vi "DEMO_07_OpenFuzhiMode.vi"() -> ()   [LabVIEW 2014]
uses:
  <vilib>/Instr/_visa.llb/VISA Configure Serial Port (Instr).vi
panel:
  in  "设置 3":bool
  in  "选择开关 3":u16(ring) items=["开始", "停止"]
  in  "选择开关 2":u16(ring) items=["开始", "停止"]
  in  "设置 2":bool
  in  "打开串口":bool
  in  "选择开关":u16(ring) items=["开始", "停止"]
  in  "上位机控制":bool
  in  "设置":bool
  in  "VISA资源名称":refnum<visa-resource-name>="COM1"
  in  "波特率":u32(ring)=9600 items=["75"=75, "110"=110, "134"=134, "150"=150, "300"=300, "600"=600, "1200"=1200, "1800"=1800, "2400"=2400, "4800"=4800, "7200"=7200, "9600"=9600, "14400"=14400, "19200"=19200, "28800"=28800, "38400"=38400, "56000"=56000, "57600"=57600, "115200"=115200, "128000"=128000, "230400"=230400]
  in  "奇偶":enum16{"None", "Odd", "Even", "Mark", "Space"}(ring) caption="校验"
  # "幅值校正控制开启"
  # "一路"
  # "二路"
  # "三路"
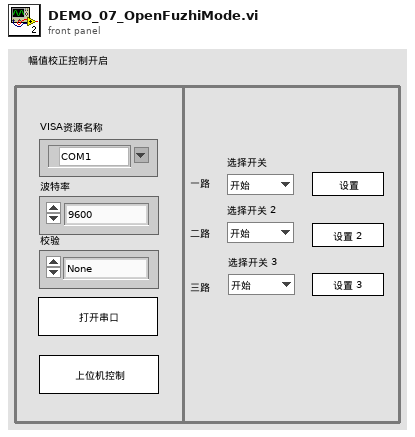
[diagram p1: front panel]
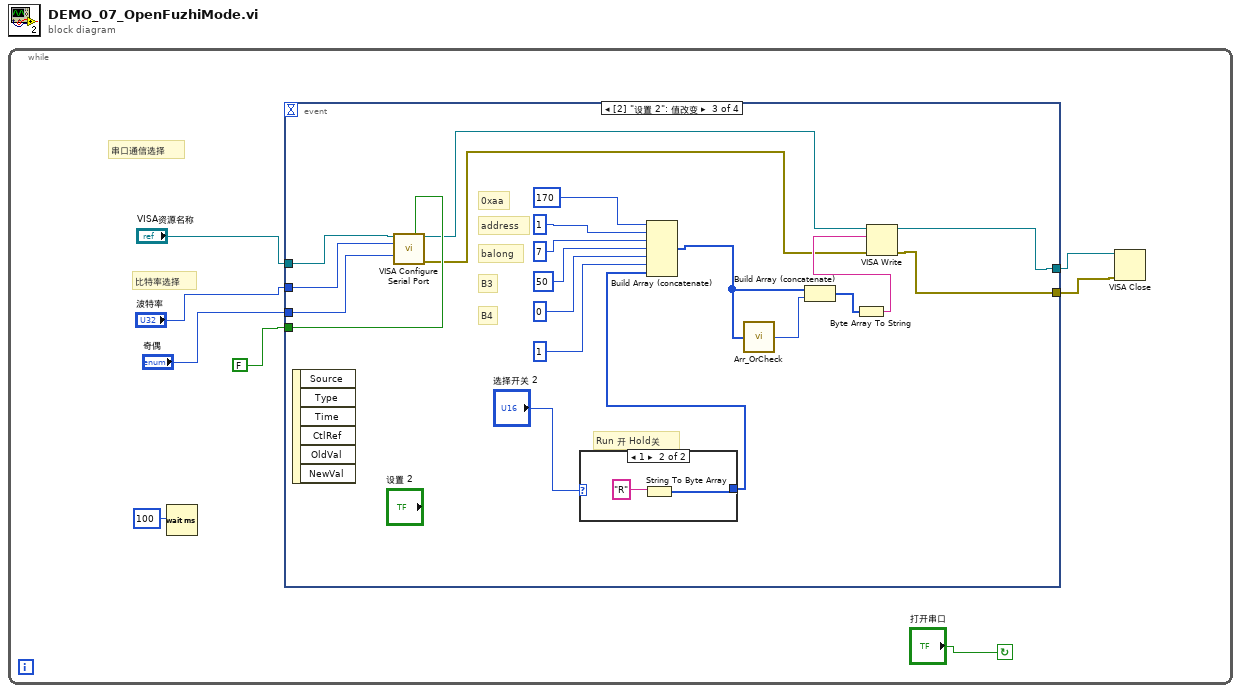
[diagram p0: block diagram]
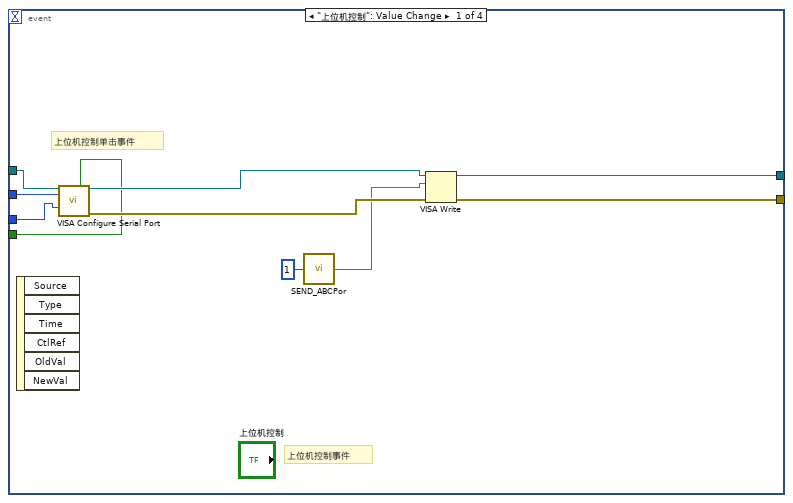
[diagram p2: hidden frame]
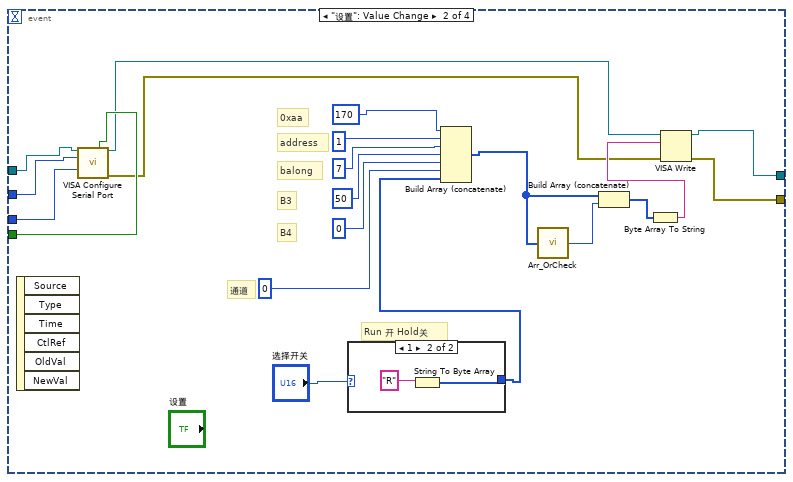
[diagram p3: hidden frame]
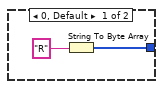
[diagram p4: hidden frame]
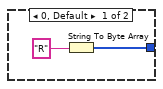
[diagram p5: hidden frame]
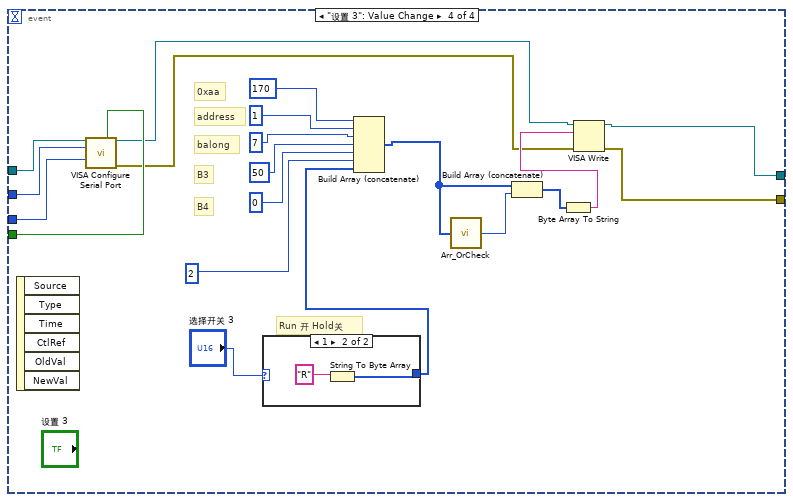
[diagram p6: hidden frame]
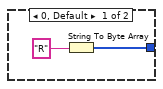
[diagram p7: hidden frame]
diagram:
  n1 = while {
    stop <- "打开串口" continue-if-true
    # "比特率选择"
    # "串口通信选择"
    n2 = Wait (ms)(milliseconds to wait=100) -> ()  [unwired: 1 out]
    n3 = event shown="[2] \"设置 2\": 值改变" {
      selector: _ -> [_ _ _ _]
      dyn-events: _ -> [_ _ _ _]
      timeout: _ -> [_ _ _ _]
      tunnel: "VISA资源名称" -> [w18 w38 w50 w76]
      tunnel: "波特率" -> [w17 w37 w49 w75]
      tunnel: "奇偶" -> [w16 w36 w48 w74]
      tunnel: [w13 w21 w44 w69] -> w1
      tunnel: [w12 w22 w43 w70] -> w6
      tunnel: FALSE -> [w11 w30 w47 w73]
      event "上位机控制": Value Change {
        # "上位机控制事件"
        # "上位机控制单击事件"
        n4 = event-data() -> ()  [unwired: 1 in, 6 out]
        n5 = call-poly "VISA Configure Serial Port"("VISA resource name"=w18, "Enable Termination\nChar (T)"=w11, "baud rate (9600)"=w17, "parity (0:none)"=w16) -> ("VISA resource name out"=w15:refnum<visa-resource-name>, "error out"=w14:errorcluster)  [unwired: 10 in]
        n6 = call "SEND_ABCPor.vi"("设备地址 1 开始"=1) -> ("输出字符串"=w9:string)
        n7 = VISA Write(VISA resource name=w15, write buffer=w9, error in (no error)=w14) -> (VISA resource name out=w13:refnum<visa-resource-name>, error out=w12:errorcluster)  [unwired: 1 out]
      }
      event "设置": Value Change {
        # "通道"
        # "B4"
        # "B3"
        # "Run 开 Hold关"
        # "balong"
        # "address"
        # "0xaa"
        n8 = event-data() -> ()  [unwired: 1 in, 6 out]
        n9 = call-poly "VISA Configure Serial Port"("VISA resource name"=w38, "Enable Termination\nChar (T)"=w30, "baud rate (9600)"=w37, "parity (0:none)"=w36) -> ("VISA resource name out"=w24:refnum<visa-resource-name>, "error out"=w23:errorcluster)  [unwired: 10 in]
        n10 = case shown="1" "选择开关" {
          tunnel: [w39 w41] -> w27
          frame 0, Default {
            n11 = String To Byte Array(string="R") -> (unsigned byte array=w39:u8[])
          }
          frame 1 {
            n12 = String To Byte Array(string="R") -> (unsigned byte array=w41:u8[])
          }
        }
        n13 = Build Array (concatenate)(170, 1, 7, 50, 0, 0 ("元素"), w27) -> (w26:i32[])
        n14 = call "Arr_OrCheck.vi"("数组"=w26) -> ("抑或的数据值"=w32:u8)
        n15 = Build Array (concatenate)(w26, w32) -> (w31:i32[])
        n16 = Byte Array To String(unsigned byte array=w31) -> (string=w25:string)
        n17 = VISA Write(VISA resource name=w24, write buffer=w25, error in (no error)=w23) -> (VISA resource name out=w21:refnum<visa-resource-name>, error out=w22:errorcluster)  [unwired: 1 out]
      }
      event "设置 2": Value Change {
        # "Run 开 Hold关"
        # "B4"
        # "B3"
        # "balong"
        # "address"
        # "0xaa"
        n18 = event-data() -> ()  [unwired: 1 in, 6 out]
        n19 = call-poly "VISA Configure Serial Port"("VISA resource name"=w50, "Enable Termination\nChar (T)"=w47, "baud rate (9600)"=w49, "parity (0:none)"=w48) -> ("VISA resource name out"=w46:refnum<visa-resource-name>, "error out"=w45:errorcluster)  [unwired: 10 in]
        n20 = case shown="1" "选择开关 2" {
          tunnel: [w63 w65] -> w52
          frame 0, Default {
            n21 = String To Byte Array(string="R") -> (unsigned byte array=w63:u8[])
          }
          frame 1 {
            n22 = String To Byte Array(string="R") -> (unsigned byte array=w65:u8[])
          }
        }
        n23 = Build Array (concatenate)(170, 1, 7, 50, 0, 1 ("元素"), w52) -> (w60:i32[])
        n24 = call "Arr_OrCheck.vi"("数组"=w60) -> ("抑或的数据值"=w62:u8)
        n25 = Build Array (concatenate)(w60, w62) -> (w61:i32[])
        n26 = Byte Array To String(unsigned byte array=w61) -> (string=w59:string)
        n27 = VISA Write(VISA resource name=w46, write buffer=w59, error in (no error)=w45) -> (VISA resource name out=w44:refnum<visa-resource-name>, error out=w43:errorcluster)  [unwired: 1 out]
      }
      event "设置 3": Value Change {
        # "Run 开 Hold关"
        # "B4"
        # "B3"
        # "balong"
        # "address"
        # "0xaa"
        n28 = event-data() -> ()  [unwired: 1 in, 6 out]
        n29 = call-poly "VISA Configure Serial Port"("VISA resource name"=w76, "Enable Termination\nChar (T)"=w73, "baud rate (9600)"=w75, "parity (0:none)"=w74) -> ("VISA resource name out"=w72:refnum<visa-resource-name>, "error out"=w71:errorcluster)  [unwired: 10 in]
        n30 = case shown="1" "选择开关 3" {
          tunnel: [w87 w89] -> w77
          frame 0, Default {
            n31 = String To Byte Array(string="R") -> (unsigned byte array=w87:u8[])
          }
          frame 1 {
            n32 = String To Byte Array(string="R") -> (unsigned byte array=w89:u8[])
          }
        }
        n33 = Build Array (concatenate)(170, 1, 7, 50, 0, 2, w77) -> (w84:i32[])
        n34 = call "Arr_OrCheck.vi"("数组"=w84) -> ("抑或的数据值"=w86:u8)
        n35 = Build Array (concatenate)(w84, w86) -> (w85:i32[])
        n36 = Byte Array To String(unsigned byte array=w85) -> (string=w83:string)
        n37 = VISA Write(VISA resource name=w72, write buffer=w83, error in (no error)=w71) -> (VISA resource name out=w69:refnum<visa-resource-name>, error out=w70:errorcluster)  [unwired: 1 out]
      }
    }
    n38 = VISA Close(VISA resource name=w1, error in (no error)=w6) -> ()  [unwired: 1 out]
  }
